vi "Lockin.DAQ.Start.vi"(8 "error in":errorcluster, 11 "Lockin.DAQ in":refnum<class "Lockin.DAQ.lvclass">) -> (0 "error out":errorcluster, 3 "Lockin.DAQ out":refnum<class "Lockin.DAQ.lvclass">)   [LabVIEW 2016, in "Lockin.DAQ.lvclass"]
uses:
  Lockin.DAQ.lvclass
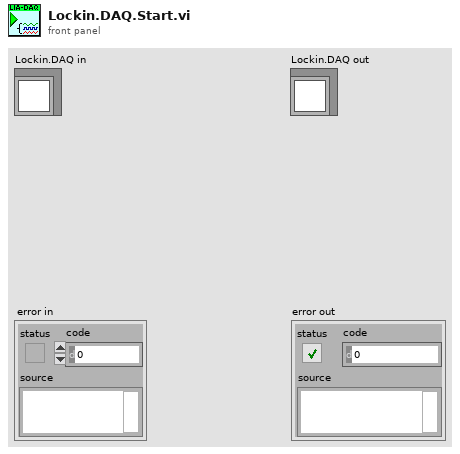
[diagram p1: front panel]
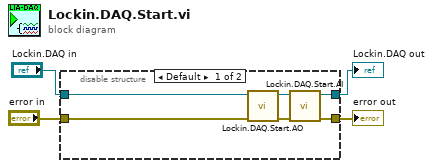
[diagram p0: block diagram]
diagram:
  n1 = disable-structure shown="Default" {
    disable-tunnel: "Lockin.DAQ in" -> [w6 w12]
    disable-tunnel: "error in" -> [w5 w11]
    disable-tunnel: [w8 w12] -> w2
    disable-tunnel: [w7 w11] -> w1
    frame condition #0 (active) {
      n2 = call "Lockin.DAQ.Start.AO.vi"("error in (no error)"=w5, "Lockin.DAQ in"=w6) -> ("error out"=w10:errorcluster, "Lockin.DAQ out"=w9:refnum<class "Lockin.DAQ.lvclass">)  [unwired: 8 in]
      n3 = call "Lockin.DAQ.Start.AI.vi"("error in (no error)"=w10, "Lockin.DAQ in"=w9) -> ("error out"=w7:errorcluster, "Lockin.DAQ out"=w8:refnum<class "Lockin.DAQ.lvclass">)  [unwired: 6 in]
    }
    frame condition #1 {
    }
  }
  "error out" <- w1
  "Lockin.DAQ out" <- w2
